vi "Example_Replay.vi"() -> ()   [LabVIEW 2015]
uses:
  TronviewGame/GameRecorder/GameRecorder.lvclass/GameRecorder.ctl
  TronviewGame/GameRecorder/GetInitialBoard.vi
  TronviewGame/GameRecorder/GetPlayer1Name.vi
  TronviewGame/GameRecorder/GetPlayer1Moves.vi
  TronviewGame/GameRecorder/GetPlayer2Name.vi
  TronviewGame/GameRecorder/GetPlayer2Moves.vi
  TronviewGame/Board/Board.lvclass
  TronviewGame/GameRecorder/GameRecorder.lvclass
  TronviewGame/TronviewGame.lvlib
  TronviewGame/Player/Player.lvclass
  ExampleBots/ReplayBot/ReplayBot.lvlib
panel:
  in  "Game string":string="p1;p2;16,16,0,0,0,0,0,0,0,0,0,0,0,0,0,0,0,0,0,0,0,0,0,0,0,0,0,0,0,0,0,0,0,0,0,0,2,0,0,0,0,0,0,0,0,0,0,0,0,0,0,0,0,0,0,0,0,0,0,0,0,0,0,0,0,0,0,0,0,0,0,0,0,0,0,0,0,0,0,0,0,0,0,0,0,0,0,0,0,0,0,0,0,0,0,0,0,0,0,0,0,0,0,0,0,0,0,0,0,0,0,0,0,0,0,0,0,0,0,0,0,0,0,0,0,0,0,0,0,0,0,0,0,0,0,0,0,0,0,0,0,0,0,0,0,0,0,0,0,0,0,0,0,0,0,0,0,0,0,0,0,0,0,0,0,0,0,0,0,0,0,0,0,0,0,0,0,0,0,0,0,0,0,0,0,0,0,0,0,0,0,0,0,0,0,0,0,0,0,0,0,0,0,0,0,0,0,0,0,0,0,0,0,0,0,0,0,0,0,0,0,0,0,0,0,0,0,0,0,0,0,0,0,0,0,0,0,0,0,0,3,0,0,0,0,0,0,0,0,0,0,0,0,0,0,0,0,0;S,S,S,E,S,W,S,W,N,W,S,S,E,E,S,S,E,N,E,N,E,S,E,S,S,S,E,E,S,W,W,W,W,N,W,W,W,S,W,N,N,E,E,E,E,E,S,S;S,E,N,N,W,W,S,S,W,W,W,W,W,W,W,W,W,W,W,W,W,N,E,E,E,E,E,E,E,E,E,E,E,E,N,W,W,W,N,E,E,E,E,E,E,N,W,W\r\n"
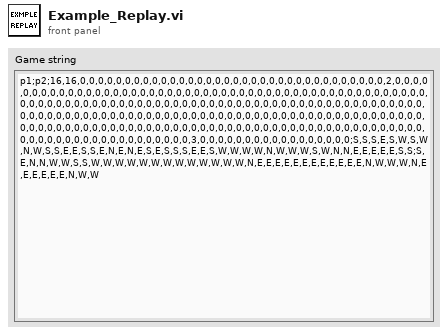
[diagram p1: front panel]
types:
  T1 = typedef "TronVIEWBotAPI.lvlib/MovementDirection.ctl" = enum16{"N", "S", "W", "E"}
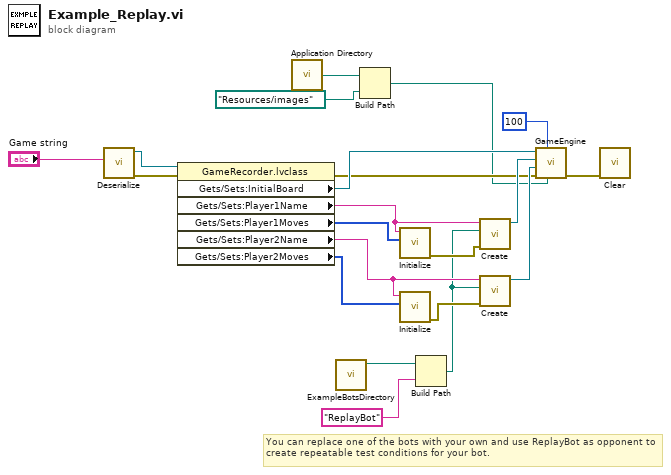
[diagram p0: block diagram]
diagram:
  # "You can replace one of the bots with your own and use ReplayBot as opponent to create repeatable test conditions for your bot."
  n1 = call "Deserialize.vi"("String"="Game string") -> ("error out"=w19:errorcluster, "GameRecorder out"=w20:refnum<class "GameRecorder.lvclass">)  [unwired: 9 in]
  n2 = property class="GameRecorder.lvclass"(reference=w20, error in=w19) -> (error out=w5:errorcluster, "Gets/Sets:InitialBoard"=w18:refnum<class "Board.lvclass">, "Gets/Sets:Player1Name"=w17:string, "Gets/Sets:Player1Moves"=w16:T1[], "Gets/Sets:Player2Name"=w13:string, "Gets/Sets:Player2Moves"=w12:T1[])  [unwired: 1 out]
  n3 = call <vilib>:"Application Directory.vi"() -> ("Application Directory"=w3:path)
  n4 = call "ExampleBotsDirectory.vi"() -> ("stripped path"=w8:path)  [unwired: 11 in]
  n5 = Build Path(base path=w3, name or relative path=path "Resources/images") -> (appended path=w1:path)
  n6 = call "Initialize.vi"("PlayerMoves"=w16, "PlayerName"=w17) -> ("error out"=w15:errorcluster)  [unwired: 9 in]
  n7 = call "Initialize.vi"("PlayerMoves"=w12, "PlayerName"=w13) -> ("error out"=w14:errorcluster)  [unwired: 9 in]
  n8 = Build Path(base path=w8, name or relative path="ReplayBot") -> (appended path=w6:path)
  n9 = call "Create.vi"("error in (no error)"=w15, "PlayerFolder"=w6, "PlayerName"=w17) -> ("Player out"=w10:refnum<class "Player.lvclass">)  [unwired: 7 in, 1 out]
  n10 = call "Create.vi"("error in (no error)"=w14, "PlayerFolder"=w6, "PlayerName"=w13) -> ("Player out"=w11:refnum<class "Player.lvclass">)  [unwired: 7 in, 1 out]
  n11 = call "GameEngine.vi"("ImagesFolder"=w1, "IterationDelay (ms)"=u32 100 ("Delay"), "error in (no error)"=w5, "Player2"=w11, "Player1"=w10, "Board"=w18) -> ("error out"=w9:errorcluster)  [unwired: 3 in, 2 out]
  n12 = call "Clear.vi"("error in (no error)"=w9) -> ()  [unwired: 10 in, 1 out]
